vi "Write Ref.vi"(8 "error in (no error)":errorcluster, 10 "Ref":u32, 11 "OSA200 in":refnum<class "OSA200.lvclass">) -> (0 "error out":errorcluster, 3 "OSA200 out":refnum<class "OSA200.lvclass">)   [LabVIEW 2010, in "OSA200.lvclass"]
uses:
  OSA200.lvclass
  OSA200.lvclass/OSA200.ctl
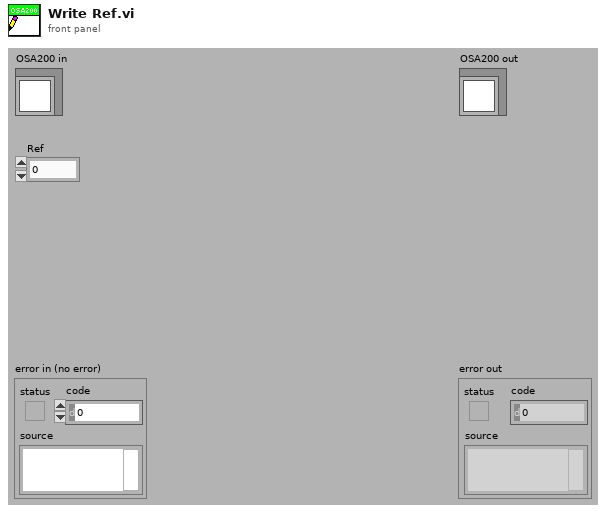
[diagram p1: front panel]
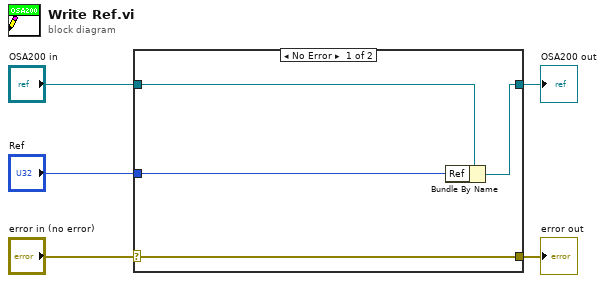
[diagram p0: block diagram]
diagram:
  n1 = case shown="No Error" "error in (no error)" {
    selector: "error in (no error)" -> [w9 w10]
    tunnel: [w9 w10] -> w4
    tunnel: [w7 w11] -> w2
    tunnel: "OSA200 in" -> [w8 w11]
    tunnel: "Ref" -> [w6 _]
    frame No Error {
      n2 = Bundle By Name(cluster=w8, "Ref"=w6) -> (w7:refnum<class "OSA200.lvclass">)
    }
    frame Error {
    }
  }
  "error out" <- w4
  "OSA200 out" <- w2
